vi "Finish Temperature.vi"(8 "error in (no error)":errorcluster, 11 "XML Handler in":refnum<class "XML Handler.lvclass">) -> (0 "error out":errorcluster, 3 "XML Handler out":refnum<class "XML Handler.lvclass">)   [LabVIEW 2020, in "XML Handler.lvclass"]
doc: "Adds the temperature to the first element of the XML document.\nIt also closes the current temperature reference."
uses:
  XML Handler.lvclass
  XML Handler.lvclass/XML Handler.ctl
  <vilib>/xml/Close Reference(Node).vi
  <vilib>/xml/NI_XML.lvlib
  <resource>/objmgr/DOMUserDefRef.rc
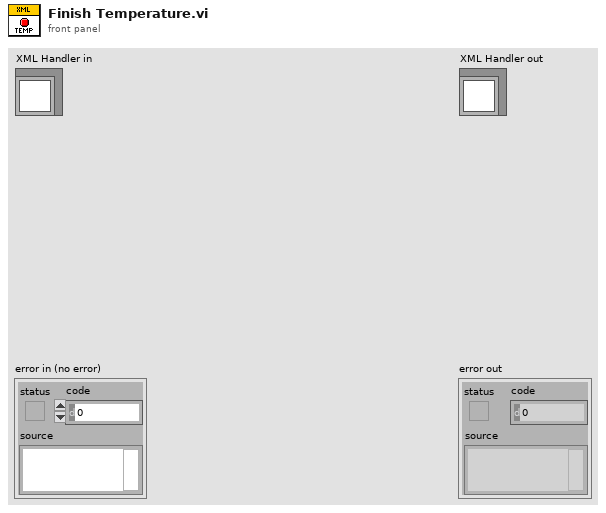
[diagram p1: front panel]
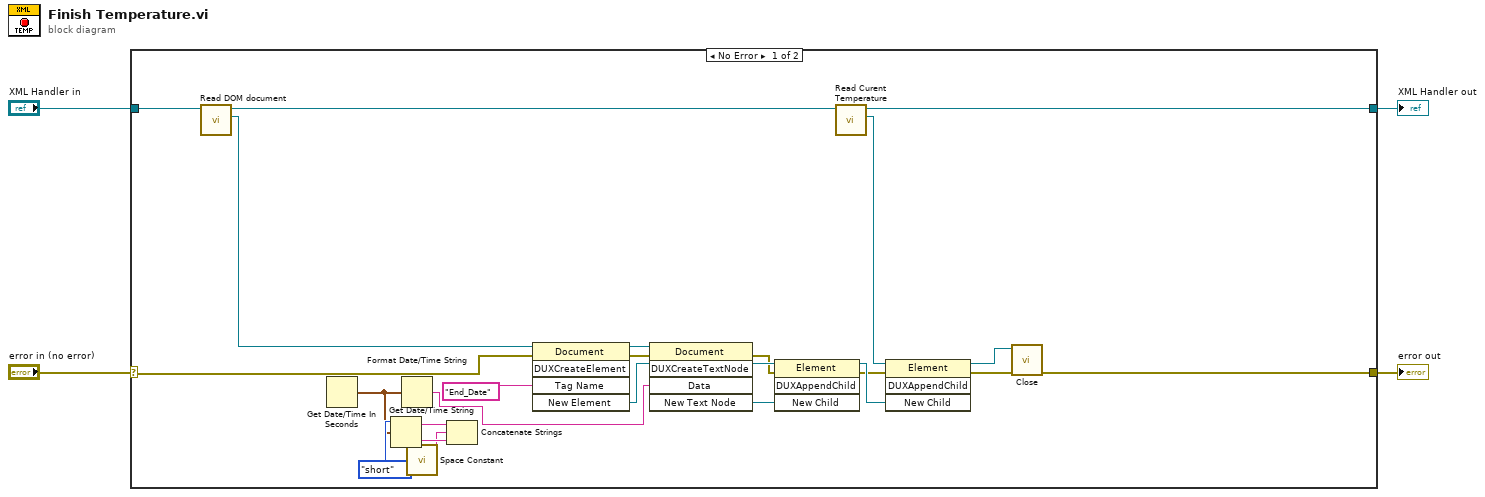
[diagram p0: block diagram]
diagram:
  n1 = case shown="No Error" "error in (no error)" {
    selector: "error in (no error)" -> [w9 w29]
    tunnel: [w10 w29] -> w3
    tunnel: [w27 w28] -> w1
    tunnel: "XML Handler in" -> [w7 w28]
    frame No Error {
      n2 = call "Read DOM document.vi"("XML Handler in"=w7) -> ("DOM document"=w8:refnum<k20>, "XML Handler out"=w6:refnum<class "XML Handler.lvclass">)  [unwired: 9 in]
      n3 = Get Date/Time In Seconds() -> (seconds since 1Jan1904=w20:timestamp)
      n4 = Get Date/Time String(date format (0)=enum16{"short", "long", "abbreviated"}."short", seconds (now)=w20) -> (date string=w24:string, time string=w23:string)  [unwired: 1 in]
      n5 = Format Date/Time String(seconds (now)=w20) -> (date/time string=w5:string)  [unwired: 2 in]
      n6 = call <vilib>:"Space Constant.vi"() -> ("String"=w22:string)
      n7 = Concatenate Strings(w24, w22, w23) -> ()  [unwired: 1 out]
      n8 = invoke class="Document" method="DUXCreateElement"(reference=w8, error in=w9, "Tag Name"="End_Date") -> (reference out=w19:refnum<k20>, error out=w18:errorcluster, "New Element"=w25:refnum<k20>)  [unwired: 2 in, 2 out]
      n9 = invoke class="Document" method="DUXCreateTextNode"(reference=w19, error in=w18, "Data"=w5) -> (error out=w17:errorcluster, "New Text Node"=w16:refnum<k20>)  [unwired: 2 in, 3 out]
      n10 = invoke class="Element" method="DUXAppendChild"(reference=w25, error in=w17, "New Child"=w16) -> (reference out=w15:refnum<k20>, error out=w14:errorcluster)  [unwired: 1 in, 2 out]
      n11 = call "Read Curent Temperature.vi"("XML Handler in"=w6) -> ("Curent Temperature"=w11:refnum<k20>, "XML Handler out"=w27:refnum<class "XML Handler.lvclass">)  [unwired: 9 in]
      n12 = invoke class="Element" method="DUXAppendChild"(reference=w11, error in=w14, "New Child"=w15) -> (reference out=w13:refnum<k20>, error out=w12:errorcluster)  [unwired: 1 in, 2 out]
      n13 = call-poly <vilib>:"Close.vi"("error in (no error)"=w12, "node"=w13) -> ("error out"=w10:errorcluster)  [unwired: 7 in]
    }
    frame Error {
    }
  }
  "error out" <- w3
  "XML Handler out" <- w1
